vi "waitForNewImages.vi"(8 "error in (no error)":errorcluster, 10 "stop":bool, 11 "AndorIKonAcquisitor in":refnum<class "AndorIKonAcquisitor.lvclass">) -> (0 "error out":errorcluster, 2 "IndexOfNewImages":i32, 3 "AndorIKonAcquisitor out":refnum<class "AndorIKonAcquisitor.lvclass">)   [LabVIEW 2009, in "Hardware.lvlib" / "Channels.lvlib" / "AndorIKonAcquisitor.lvclass"]
uses:
  AndorIKonAcquisitor.lvclass
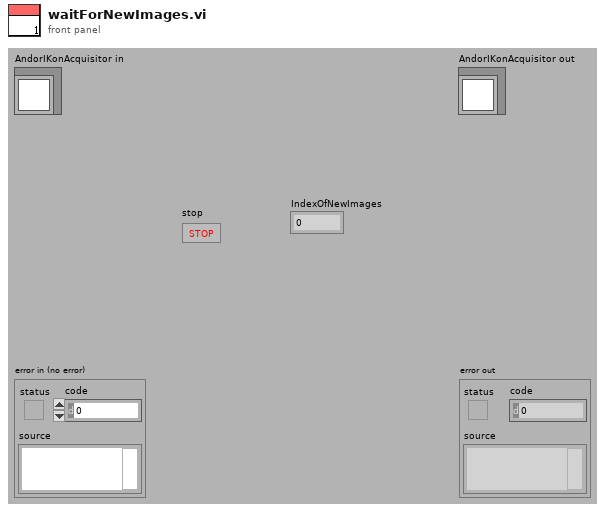
[diagram p1: front panel]
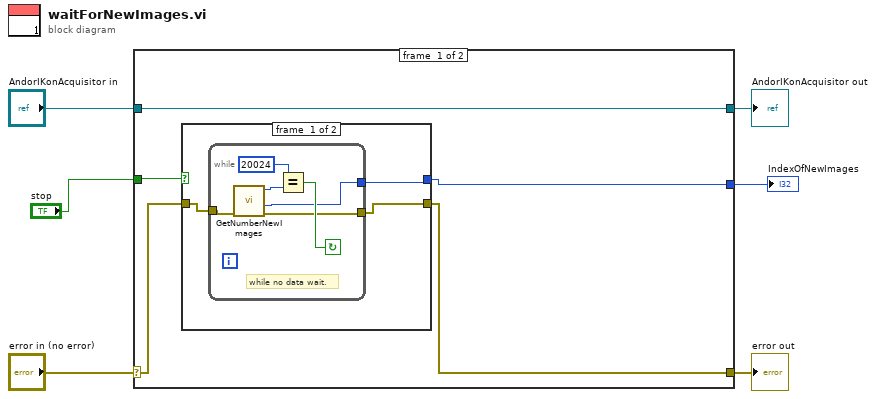
[diagram p0: block diagram]
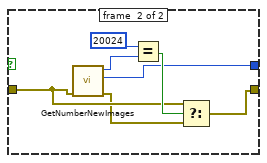
[diagram p2: hidden frame]
diagram:
  n1 = case shown="No Error" "error in (no error)" {
    selector: "error in (no error)" -> [w11 w29]
    tunnel: [w10 w29] -> w5
    tunnel: [w9 w28] -> w3
    tunnel: "AndorIKonAcquisitor in" -> [w9 w28]
    tunnel: "stop" -> [w8 _]
    tunnel: [w7 _] -> w1
    frame #0 {
      n2 = case shown="False" w8 {
        tunnel: w11 -> [w14 w24]
        tunnel: [w13 w22] -> w10
        tunnel: [w12 w21] -> w7
        frame #0 {
          n3 = while {
            tunnel: w14 -> [w20]
            tunnel: [w16] -> w13
            tunnel: [w15] -> w12
            stop <- w17 continue-if-true
            # "while no data wait."
            n4 = call <userlib>:"GetNumberNewImages.vi"("error in (no error)"=w20) -> ("error out"=w16:errorcluster, "last"=w15:i32, "DLL error code"=w18:u32)  [unwired: 3 in, 1 out]
            n5 = Equal?(x=20024, y=w18) -> (x = y?=w17:bool)
          }
        }
        frame #1 {
          n6 = call <userlib>:"GetNumberNewImages.vi"("error in (no error)"=w24) -> ("error out"=w23:errorcluster, "first"=w21:u32, "DLL error code"=w26:u32)  [unwired: 3 in, 1 out]
          n7 = Equal?(x=20024, y=w26) -> (x = y?=w25:bool)
          n8 = Select(t=w24, s=w25, f=w23) -> (s? t:f=w22:errorcluster)
        }
      }
    }
    frame #1 {
    }
  }
  "error out" <- w5
  "AndorIKonAcquisitor out" <- w3
  "IndexOfNewImages" <- w1
